vi "VoltageUpdate.Read Configuration File.vi"(8 "error in (no error)":errorcluster, 11 "VoltageUpdate":refnum<class "VoltageUpdate.lvclass">) -> (0 "error out":errorcluster, 3 "VoltageUpdate out":refnum<class "VoltageUpdate.lvclass">)   [LabVIEW 2016, in "VoltageUpdate.lvclass"]
uses:
  VoltageUpdate.lvclass
  C:/Program Files (x86)/National Instruments/LabVIEW 2016/user.lib/LevyLab/Levylab Instruments/SMOs/Instrument/Instrument.lvclass
  VoltageUpdate.lvclass/VoltageUpdate.ctl
  <userlib>/LevyLab/Levylab Instruments/SMOs/Instrument/Instrument.lvclass/Instrument.ctl
  <userlib>/LevyLab/Levylab Instruments/SMOs/Configuration/Configuration.lvclass
  <userlib>/LevyLab/Levylab Instruments/SMOs/Instrument/Instrument.lvclass
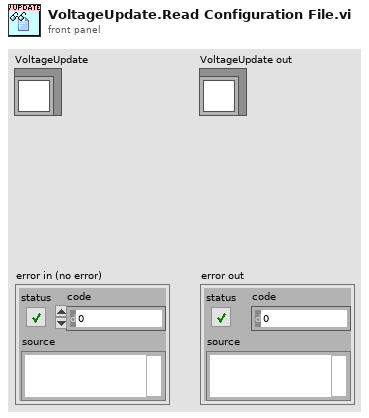
[diagram p1: front panel]
types:
  T1 = typedef "VoltageUpdate.lvclass/VoltageUpdate.Configuration--Cluster.ctl" = cluster{"Amplfier Gain":dbl}
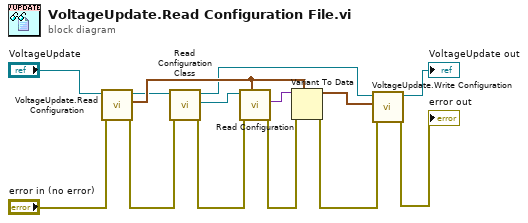
[diagram p0: block diagram]
diagram:
  n1 = call "VoltageUpdate.Read Configuration.vi"("error in (no error)"="error in (no error)", "VoltageUpdate"="VoltageUpdate") -> ("error out"=w6:errorcluster, "Configuration"=w10:T1, "VoltageUpdate out"=w8:refnum<class "VoltageUpdate.lvclass">)  [unwired: 7 in]
  n2 = call <userlib>:"Read Configuration Class.vi"("error in (no error)"=w6, "Instrument in"=w8) -> ("error out"=w5:errorcluster, "Configuration.lvclass"=w9:refnum<class "Configuration.lvclass">, "Instrument out"=w7:refnum<class "VoltageUpdate.lvclass">)  [unwired: 7 in]
  n3 = call <userlib>:"Read Configuration.vi"("INI Fomatted Cluster Type"=w10, "error in (no error)"=w5, "Configuration in"=w9) -> ("error out"=w13:errorcluster, "Configuration"=w14:variant)  [unwired: 6 in, 1 out]
  n4 = Variant To Data(error in=w13, type=w10, Variant=w14) -> (data=w12:T1, error out=w11:errorcluster)
  n5 = call "VoltageUpdate.Write Configuration.vi"("error in (no error)"=w11, "Configuration"=w12, "VoltageUpdate"=w7) -> ("error out"=→"error out":errorcluster, "VoltageUpdate out"=→"VoltageUpdate out":refnum<class "VoltageUpdate.lvclass">)  [unwired: 7 in]
